vi "Create Instance Impl.vi"(8 "error in (no error)":errorcluster, 10 "Stage Configuration":T1={"Serial Port"="COM4", "Forward Step (mm)"=0.4, "Lane Length (mm)"=6.0, "Lane Separation (mm)"=0.8, "Stage Type"=enum."Ti2", "Autofocus Z Planes"=9, "Autofocus Range (um)"=30.0, "Stage Limits"={"Y Min"=-4.5, "Y Max"=3.0, "X Min"=-19.0, "X Max"=33.5}, "Slide (mm)"={"top"=-13.0, "right"=-22.3, "width"=60.0, "height"=25.4}}, 11 "ASI Stage in":refnum<class "ASI Stage.lvclass">) -> (0 "error out":errorcluster, 3 "ASI Stage out":refnum<class "ASI Stage.lvclass">)   [LabVIEW 2023, in "ASI Stage.lvlib" / "ASI Stage.lvclass"]
uses:
  Resources/Type Defs/Stage Configuration.ctl
  ASI Stage.lvclass
  ASI Stage.lvclass/ASI Stage.ctl
  <instrlib>/ASI TG-1000/ASI TG-1000.lvlib
  <instrlib>/ASI TG-1000/Public/Utility/Baud Rate.ctl
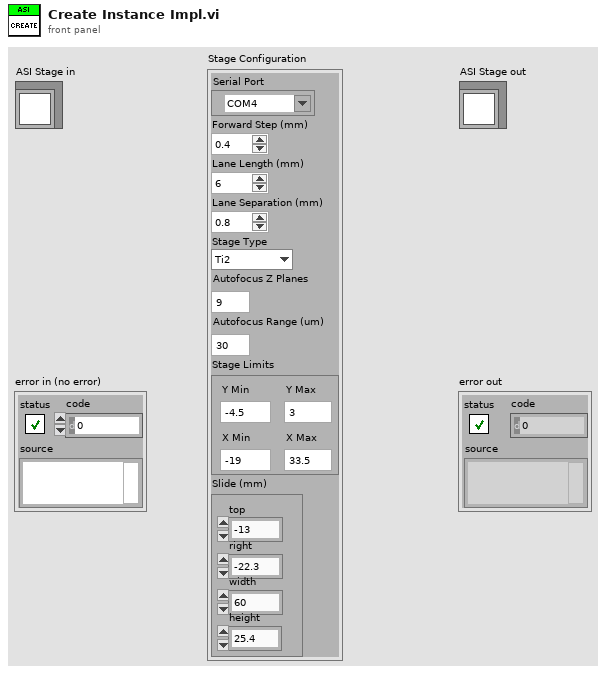
[diagram p1: front panel]
types:
  T1 = typedef "Stage Configuration.ctl" = cluster{"Serial Port":refnum<visa-resource-name>, "Forward Step (mm)":dbl, "Lane Length (mm)":dbl, "Lane Separation (mm)":dbl, "Stage Type":enum16{"Disabled", "ESP301", "Ti2", "Ludl", "ASI"}, "Autofocus Z Planes":i32, "Autofocus Range (um)":dbl, "Stage Limits":cluster{"Y Min":dbl, "Y Max":dbl, "X Min":dbl, "X Max":dbl}, "Slide (mm)":cluster{"top":dbl, "right":dbl, "width":dbl, "height":dbl}}
  T2 = typedef "ASI TG-1000.lvlib/Baud Rate.ctl" = u32
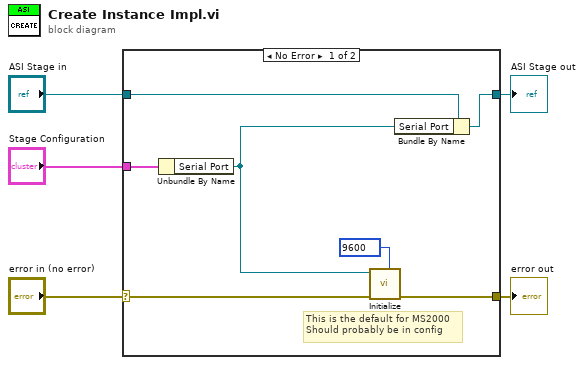
[diagram p0: block diagram]
diagram:
  n1 = case shown="No Error" "error in (no error)" {
    selector: "error in (no error)" -> [w10 w14]
    tunnel: [w11 w14] -> w5
    tunnel: "Stage Configuration" -> [w7 _]
    tunnel: "ASI Stage in" -> [w9 w13]
    tunnel: [w8 w13] -> w1
    frame No Error {
      w12 = T2 9600 items=["9600"=9600, "19200"=19200, "28800"=28800, "115200"=115200] ("Baud Rate (115200)")
      # "This is the default for MS2000\nShould probably be in config"
      n2 = Unbundle By Name(w7) -> ("Serial Port"=w6:refnum<visa-resource-name>)
      n3 = call <instrlib>:"Initialize.vi"("Baud Rate (115200)"=w12, "error in (no error)"=w10, "VISA resource name"=w6) -> ("error out"=w11:errorcluster)  [unwired: 7 in, 1 out]
      n4 = Bundle By Name(cluster=w9, "Serial Port"=w6) -> (w8:refnum<class "ASI Stage.lvclass">)
    }
    frame Error {
    }
  }
  "error out" <- w5
  "ASI Stage out" <- w1
